vi "Write Instrument Setting.vi"(8 "error in (no error)":errorcluster, 10 "Instrument Setting":T1={"Type"="None", "Address"="localhost", "SW Alias"="Type = Class \n", "Description"="1.0.0.0", "Enabled"=TRUE}, 11 "Instrument configuration in":refnum<class "Instrument configuration.lvclass">) -> (0 "error out":errorcluster, 3 "Instrument configuration out":refnum<class "Instrument configuration.lvclass">)   [LabVIEW 2025, in "Abstract Engine.lvlib" / "Instrument configuration.lvclass"]
uses:
  Instrument configuration.lvclass
  Instrument configuration.lvclass/Instrument configuration.ctl
  Default Instrument.ctl
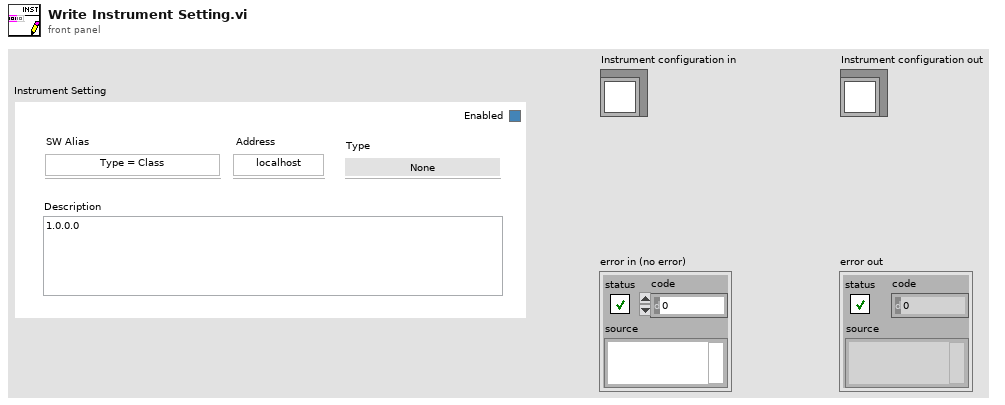
[diagram p1: front panel]
types:
  T1 = typedef "Abstract Engine.lvlib/Instrument configuration.lvclass/Default Instrument.ctl" = cluster{"Type":string, "Address":string, "SW Alias":string, "Description":string, "Enabled":bool}
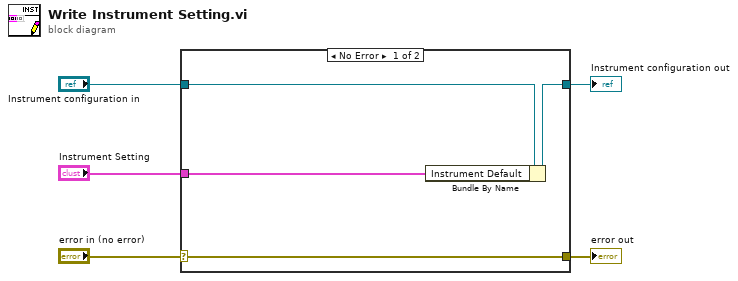
[diagram p0: block diagram]
diagram:
  n1 = case shown="No Error" "error in (no error)" {
    selector: "error in (no error)" -> [w9 w10]
    tunnel: [w9 w10] -> w4
    tunnel: [w7 w11] -> w2
    tunnel: "Instrument configuration in" -> [w8 w11]
    tunnel: "Instrument Setting" -> [w6 _]
    frame No Error {
      n2 = Bundle By Name(cluster=w8, "Instrument Default"=w6) -> (w7:refnum<class "Instrument configuration.lvclass">)
    }
    frame Error {
    }
  }
  "error out" <- w4
  "Instrument configuration out" <- w2
